vi "Build Category Menu.vi"(8 "error in (no error)":errorcluster, 10 "MenuRef":refnum<k9>, 11 "Budgetizer in":refnum<class "Budgetizer.lvclass">) -> (0 "error out":errorcluster, 3 "Budgetizer out":refnum<class "Budgetizer.lvclass">)   [LabVIEW 2018, in "Budgetizer.lvclass"]
uses:
  Budgetizer.lvclass
  Category/Category.lvclass
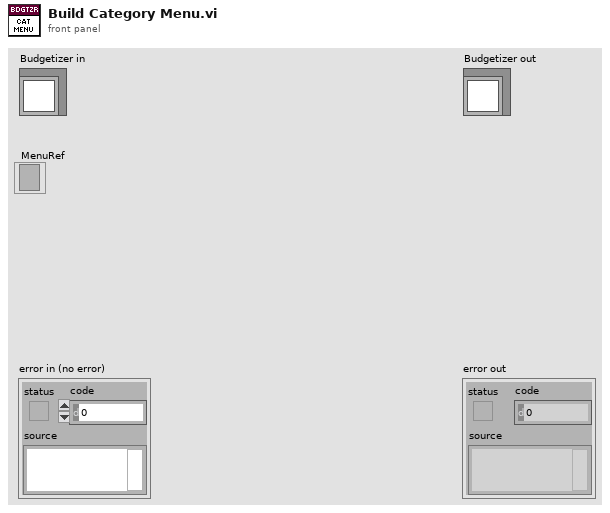
[diagram p1: front panel]
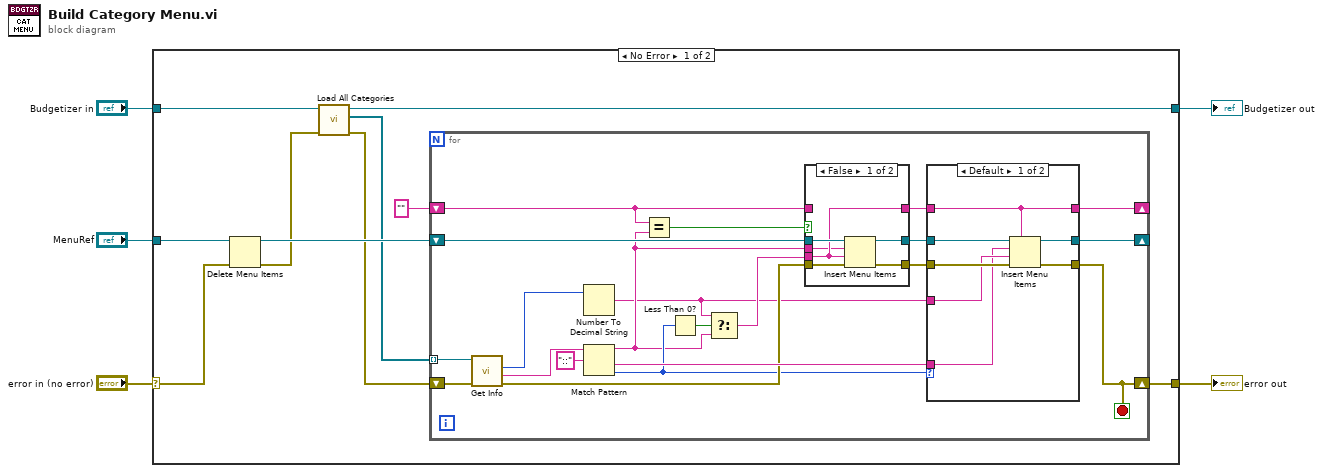
[diagram p0: block diagram]
diagram:
  n1 = case shown="No Error" "error in (no error)" {
    selector: "error in (no error)" -> [w13 w57]
    tunnel: [w14 w57] -> w4
    tunnel: [w9 w56] -> w2
    tunnel: "Budgetizer in" -> [w10 w56]
    tunnel: "MenuRef" -> [w15 _]
    frame No Error {
      n2 = Delete Menu Items(6:w13, 9:w15) -> (0:w8:errorcluster, 3:w12:refnum<k9>)  [unwired: 2 in]
      n3 = call "Load All Categories.vi"("error in (no error)"=w8, "Budgetizer in"=w10) -> ("error out"=w7:errorcluster, "Categories"=w6:refnum<class "Category.lvclass">[], "Budgetizer out"=w9:refnum<class "Budgetizer.lvclass">)  [unwired: 7 in]
      n4 = for {
        shift-right: [w34] -> w14
        shift-left: w7 -> [w27]
        shift-right: [w30] -> _
        shift-left: w12 -> [w35]
        shift-right: [w18] -> _
        shift-left: "" -> [w28]
        tunnel: w6 -> [w26] mode=indexing
        stop <- w34 stop-if-true
        n5 = call "Get Info.vi"("error in (no error)"=w27, "Category in"=w26) -> ("error out"=w25:errorcluster, "Name"=w24:string, "id"=w23:i32)  [unwired: 6 in, 1 out]
        n6 = Number To Decimal String(number=w23) -> (decimal integer string=w16:string)  [unwired: 1 in]
        n7 = Match Pattern(string=w24, regular expression="::") -> (before substring=w20:string, after substring=w32:string, offset past match=w22:i32)  [unwired: 1 in, 1 out]
        n8 = Equal?(x=w28, y=w20) -> (x = y?=w29:bool)
        n9 = Less Than 0?(x=w22) -> (x < 0?=w21:bool)
        n10 = Select(t=w16, s=w21, f=w20) -> (s? t:f=w17:string)
        n11 = case shown="False" w29 {
          tunnel: w35 -> [w42 w45]
          tunnel: w25 -> [w41 w44]
          tunnel: [w40 w44] -> w33
          tunnel: [w39 w45] -> w31
          tunnel: w20 -> [w37 _]
          tunnel: w28 -> [_ w43]
          tunnel: w17 -> [w38 _]
          tunnel: [w38 w43] -> w19
          frame False {
            n12 = Insert Menu Items(6:w41, 7:w38, 8:w37, 9:w42) -> (0:w40:errorcluster, 3:w39:refnum<k9>)  [unwired: 2 in, 1 out]
          }
          frame True {
          }
        }
        n13 = case shown="Default" w22 {
          tunnel: [w51 w55] -> w34
          tunnel: w33 -> [w52 w55]
          tunnel: w32 -> [w46 _]
          tunnel: w31 -> [w50 w54]
          tunnel: [w49 w54] -> w30
          tunnel: w19 -> [w48 w53]
          tunnel: [w48 w53] -> w18
          tunnel: w16 -> [w47 _]
          frame Default {
            n14 = Insert Menu Items(5:w48, 6:w52, 7:w47, 8:w46, 9:w50) -> (0:w51:errorcluster, 3:w49:refnum<k9>)  [unwired: 1 in, 1 out]
          }
          frame -1 {
          }
        }
      }
    }
    frame Error {
    }
  }
  "error out" <- w4
  "Budgetizer out" <- w2
